vi "NI WaitForSegs.vi"(0 "NI ID":refnum<k15>, 2 "lines per plane":u16, 3 "error in":errorcluster, 4 "Timeout":i32=5000) -> (5 "Instrument ID":refnum<k15>, 6 "status":bool, 7 "error out":errorcluster)   [LabVIEW 2022 SP3]
panel:
  out "Fetch:Records Done":i32
  out "lines acquired":i32
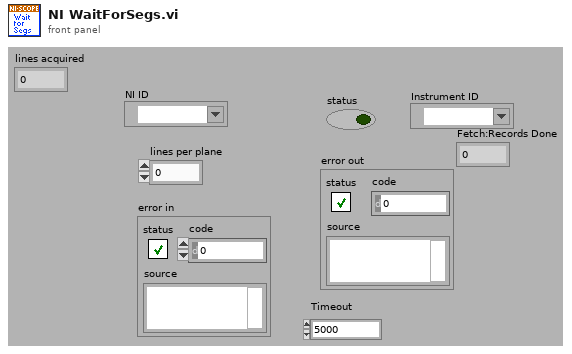
[diagram p1: front panel]
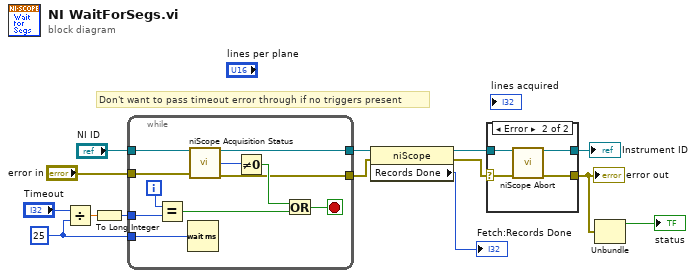
[diagram p0: block diagram]
diagram:
  w12 = u32 25 ("milliseconds to wait")
  # "Don't want to pass timeout error through if no triggers present"
  n1 = Divide(x="Timeout", y=w12) -> (x/y=w11:dbl)
  n2 = To Long Integer(number=w11) -> (32bit integer=w8:i32)
  n3 = while {
    tunnel: "NI ID" -> [w25]
    tunnel: w12 -> [w23]
    tunnel: w8 -> [w22]
    tunnel: [w17] -> w6
    tunnel: [w16] -> w7
    tunnel: "error in" -> [w15]
    i -> [w21]
    stop <- w20 stop-if-true
    n4 = Equal?(x=w21, y=w22) -> (x = y?=w19:bool)
    n5 = Wait (ms)(milliseconds to wait=w23) -> ()  [unwired: 1 out]
    n6 = call <instrlib>:"niScope Acquisition Status.vi"("instrument handle"=w25, "error in"=w15) -> ("instrument handle out"=w16:refnum<k15>, "acquisition status"=w24:i32, "error out"=w17:errorcluster)  [unwired: 11 out]
    n7 = Not Equal To 0?(x=w24) -> (x != 0?=w18:bool)
    n8 = Or(x=w18, y=w19) -> (x .or. y?=w20:bool)
  }
  n9 = property class="niScope"(reference=w7, error in=w6) -> (reference out=w4:refnum<k15>, error out=w5:errorcluster, "Records Done"=→"Fetch:Records Done":i32)
  n10 = case shown="Error" w5 {
    selector: w5 -> [w26 w30]
    tunnel: w4 -> [w27 w31]
    tunnel: [w27 w29] -> w3
    tunnel: [w26 w28] -> w2
    frame No Error {
    }
    frame Error {
      n11 = call <instrlib>:"niScope Abort.vi"("instrument handle"=w31, "error in"=w30) -> ("instrument handle out"=w29:refnum<k15>, "error out"=w28:errorcluster)  [unwired: 12 out]
    }
  }
  "error out" <- w2
  "Instrument ID" <- w3
  n12 = Unbundle(w2) -> ("status"=→"status":bool)  [unwired: 2 out]
